vi "Pre Launch Init.vi"(11 "Nested in":refnum<class "MQTT_Client_Actor.lvclass">) -> (0 "error out":errorcluster, 3 "Nested out":refnum<class "MQTT_Client_Actor.lvclass">)   [LabVIEW 2018, in "MQTT_Client_Actor.lvlib" / "MQTT_Client_Actor.lvclass"]
doc: "(<B>Filename</B>: Actor Framework.lvlib:Actor.lvclass:Pre Launch Init.vi)\n\nDefines behavior that occurs after the Launch Nested Actor method is invoked but before the actor's Actor Core method begins running.\n\nBy default, this method does nothing. A descendant class may override it to define behavior."
uses:
  MQTT_Client_Actor.lvclass
  PublishClient.ctl
  <vilib>/LabVIEW Open Source Project/MQTT Control Packets/Control Packets/ControlPacket/QualityOfService -- enum.ctl
  SubscribeClient.ctl
  CreateClient.ctl
  MQTT_Client_Actor.lvclass/MQTT_Client_Actor.ctl
  <vilib>/ActorFramework/Actor/Actor.lvclass
  <vilib>/LabVIEW Open Source Project/MQTT Control Packets/Control Packets/ControlPacket/ControlPacket.lvclass
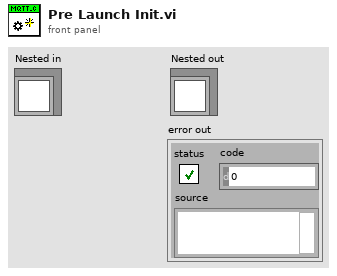
[diagram p1: front panel]
types:
  T1 = typedef "MQTT_Client_Actor.lvlib/MQTT_Client_Actor.lvclass/PublishClient.ctl" = cluster{"Topic Name":string, "QoS":T2, "RETAIN":bool, "Topic Data":string}
  T2 = typedef "MQTT_Control_Packets.lvlib/ControlPacket.lvclass/QualityOfService -- enum.ctl" = enum16{"0 (At Most Once)", "1 (At Least Once)", "2 (Exactly Once)"}
  T3 = typedef "MQTT_Client_Actor.lvlib/MQTT_Client_Actor.lvclass/SubscribeClient.ctl" = cluster{"Topic Name":string, "QoS":T2, "T:Subscribe":bool}
  T4 = typedef "MQTT_Client_Actor.lvlib/MQTT_Client_Actor.lvclass/CreateClient.ctl" = cluster{"address":string, "port":u16, "UserName":string, "Pwd":string}
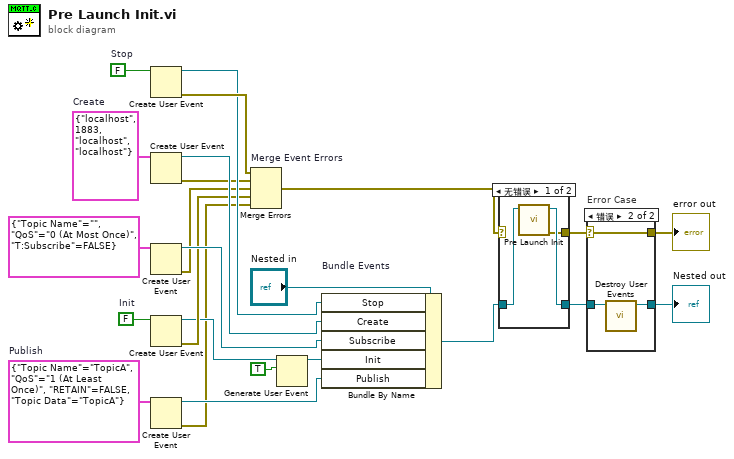
[diagram p0: block diagram]
diagram:
  w3 = T1 {"Topic Name"="TopicA", "QoS"=enum."1 (At Least Once)", "RETAIN"=FALSE, "Topic Data"="TopicA"}  # Publish
  w9 = FALSE  # Init
  w14 = T4 {"address"="localhost", "port"=1883, "UserName"="localhost", "Pwd"="localhost"}  # Create
  w23 = FALSE  # Stop
  n1 = Create User Event(user event datatype=w23) -> (user event=w20:refnum<user-event>, error out=w22:errorcluster)  [unwired: 1 in]
  n2 = Create User Event(user event datatype=w14) -> (user event=w13:refnum<user-event>, error out=w12:errorcluster)  [unwired: 1 in]
  n3 = Create User Event(user event datatype=T3 {"Topic Name"="", "QoS"=enum."0 (At Most Once)", "T:Subscribe"=FALSE} ("簇")) -> (user event=w11:refnum<user-event>, error out=w10:errorcluster)  [unwired: 1 in]
  n4 = Create User Event(user event datatype=w9) -> (user event=w6:refnum<user-event>, error out=w8:errorcluster)  [unwired: 1 in]
  n5 = Create User Event(user event datatype=w3) -> (user event=w2:refnum<user-event>, error out=w1:errorcluster)  [unwired: 1 in]
  n6 = Merge Errors "Merge Event Errors"(w22, w12, w10, w8, w1) -> (w16:errorcluster)
  n7 = Generate User Event(user event=w6, event data cluster=TRUE ("事件数据")) -> (user event out=w5:refnum<user-event>)  [unwired: 2 in, 1 out]
  n8 = Bundle By Name "Bundle Events"(cluster="Nested in", "Stop"=w20, "Create"=w13, "Subscribe"=w11, "Init"=w5, "Publish"=w2) -> (w17:refnum<class "MQTT_Client_Actor.lvclass">)
  n9 = case shown="无错误" w16 {
    selector: w16 -> [_ w29]
    tunnel: [w27 w28] -> w18
    tunnel: w17 -> [w26 w28]
    tunnel: [w25 w29] -> w15
    frame No Error {
      n10 = call-parent "Pre Launch Init.vi"("Actor in"=w26) -> ("error out"=w25:errorcluster, "Actor out"=w27:refnum<class "MQTT_Client_Actor.lvclass">)  [unwired: 9 in]
    }
    frame Error {
    }
  }
  n11 = case "Error Case" shown="错误" w15 {
    selector: w15 -> [w30 w34]
    tunnel: w18 -> [w31 w33]
    tunnel: [w31 w32] -> w21
    tunnel: [w30 w34] -> w19
    frame No Error {
    }
    frame Error {
      n12 = call "Destroy User Events.vi"("UI Template in"=w33) -> ("UI Template out"=w32:refnum<class "MQTT_Client_Actor.lvclass">)  [unwired: 10 in]
    }
  }
  "error out" <- w19
  "Nested out" <- w21
